vi "Default DateFile Path - Constant.vi"() -> (3 "Datafile Path (Default)":path)   [LabVIEW 2021]
doc: "The default filepath is \"Calibration (default).txt\", in the folder of the main VI/project file."
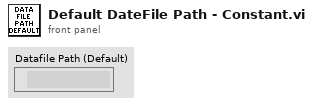
[diagram p1: front panel]
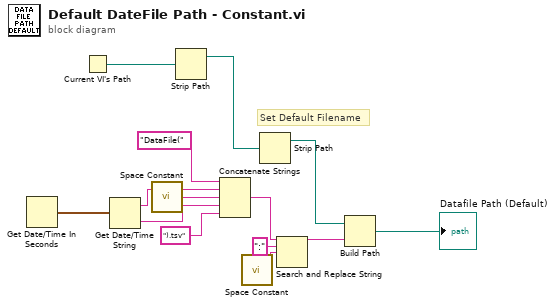
[diagram p0: block diagram]
diagram:
  # "Set Default Filename"
  n1 = Get Date/Time In Seconds() -> (seconds since 1Jan1904=w5:timestamp)
  n2 = Current VI's Path() -> (path=w2:path)
  n3 = Get Date/Time String(seconds (now)=w5) -> (date string=w7:string, time string=w9:string)  [unwired: 2 in]
  n4 = call <vilib>:"Space Constant.vi"() -> ("String"=w8:string)
  n5 = Strip Path(path=w2) -> (stripped path=w1:path)  [unwired: 1 out]
  n6 = Concatenate Strings("DataFile(" ("string"), w7, w8, w9, ").tsv" ("string")) -> (w11:string)
  n7 = call <vilib>:"Space Constant.vi"() -> ("String"=w13:string)
  n8 = Strip Path(path=w1) -> (stripped path=w3:path)  [unwired: 1 out]
  n9 = Search and Replace String(input string=w11, search string=":", replace string=w13) -> (result string=w14:string)  [unwired: 5 in, 3 out]
  n10 = Build Path(base path=w3, name or relative path=w14) -> (appended path=→"Datafile Path (Default)":path)
